vi "CAN Timeout.vi"(7 "Aktionen":T1, 8 "Fehler":errorcluster caption="Fehler (Eingang, kein Fehler)", 10 "Zeitstempel":timestamp) -> (2 "Zeitstempel":timestamp, 5 "Aktionen":T1)   [LabVIEW 2020, in "CAN Interface.lvlib"]
uses:
  CAN Interface.lvlib
  CAN Komm Aktionen.ctl
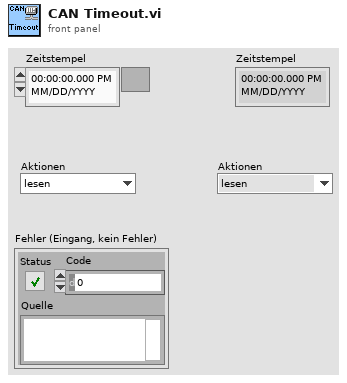
[diagram p1: front panel]
types:
  T1 = typedef "CAN Interface.lvlib/CAN Komm Aktionen.ctl" = enum16{"lesen", "init", "Komm", "beenden", "flush"}
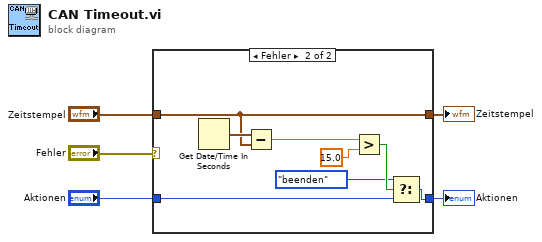
[diagram p0: block diagram]
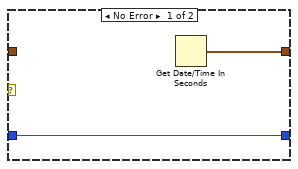
[diagram p2: hidden frame]
diagram:
  n1 = case shown="Fehler" "Fehler" {
    tunnel: [w7 w14] -> w1
    tunnel: "Zeitstempel" -> [_ w14]
    tunnel: "Aktionen" -> [w6 w11]
    tunnel: [w6 w9] -> w5
    frame No Error {
      n2 = Get Date/Time In Seconds() -> (seconds since 1Jan1904=w7:timestamp)
    }
    frame Error {
      n3 = Get Date/Time In Seconds() -> (seconds since 1Jan1904=w15:timestamp)
      n4 = Subtract(x=w15, y=w14) -> (x-y=w13:dbl)
      n5 = Greater?(x=w13, y=15.0) -> (0:w12:bool)
      n6 = Select(t=CAN_Komm_Aktionen."beenden" ("Aktionen"), s=w12, f=w11) -> (s? t:f=w9:T1)
    }
  }
  "Aktionen" <- w5
  "Zeitstempel" <- w1
